vi "Next State.vi"(2 "Buttons []":bool[](array[boolean]), 3 "States []":T1[](array[typedef])) -> (0 "Save Next?":bool, 1 "Enum":T1)   [LabVIEW 2012]
uses:
  Mega Awesome/data/MegaAwesome_States.ctl
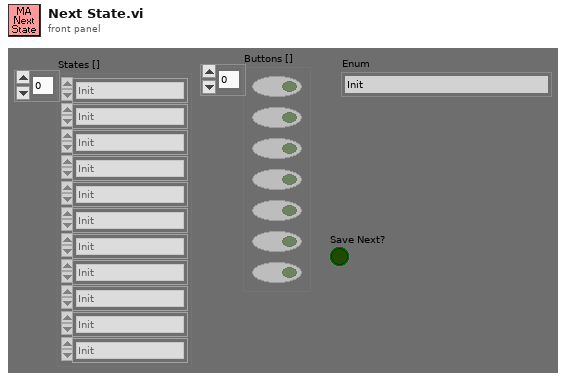
[diagram p1: front panel]
types:
  T1 = typedef "MegaAwesome_States.ctl" = enum16{"Init", "File Missing", "No Event", "Read Data", "Calculated Values", "Re-Calculated Values", "Next File", "Previous File", "Discard File", "Save", "Save Lines", "Export", "Exit"}
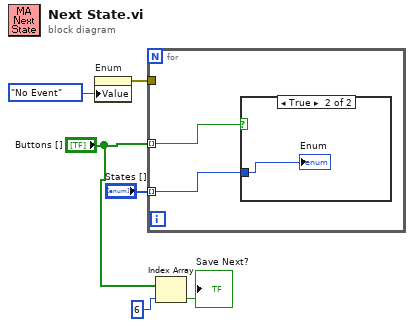
[diagram p0: block diagram]
diagram:
  n1 = property on="Enum" class="Enum (strict)"("Value"=MegaAwesome_States."No Event") -> (error out=w5:errorcluster)  [unwired: 2 in, 1 out]
  n2 = for {
    tunnel: "Buttons []" -> [w8] mode=indexing
    tunnel: "States []" -> [w7] mode=indexing
    tunnel: w5 -> [_]
    n3 = case shown="True" w8 {
      tunnel: w7 -> [_ w9]
      frame False {
      }
      frame True {
        "Enum" <- w9
      }
    }
  }
  n4 = Index Array(array="Buttons []", index=6) -> (element=→"Save Next?":bool)
